vi "VI Data Extractor.vi"(7 "Port number":u16=3364, 8 "error in (no error)":errorcluster, 10 "Output path":path, 11 "VI Path":path) -> (0 "error out":errorcluster, 3 "path":path)   [LabVIEW 2024]
uses:
  <vilib>/Utility/traverseref.llb/TRef TravTarget.ctl
  <vilib>/Utility/miscctls.llb/LVPositionTypeDef.ctl
  <vilib>/Utility/miscctls.llb/LVBoundsTypeDef.ctl
  <vilib>/Utility/miscctls.llb/LVMapReplaceAction.ctl
  <vilib>/Utility/traverseref.llb/VI Scripting - Traverse.lvlib
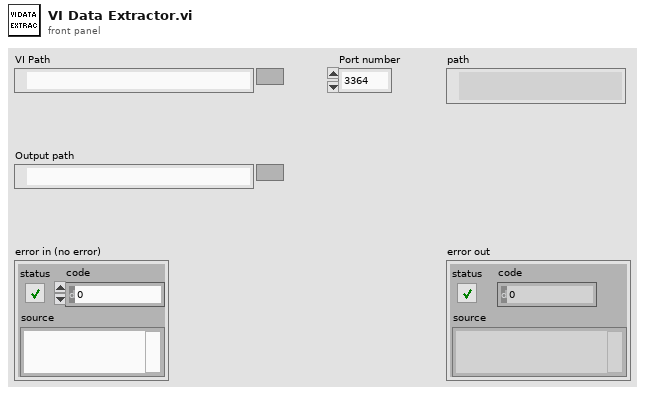
[diagram p1: front panel]
types:
  T1 = typedef "LVPositionTypeDef.ctl" = cluster{"Left":i32, "Top":i32}
  T2 = typedef "LVBoundsTypeDef.ctl" = cluster{"Width":u32, "Height":u32}
  T3 = map{i32, cluster{"Diagram Data":cluster{"UID":i32, "Diagram Image":string}[], "Position":T1, "Bounds":T2, "Is on TLD?":bool}}
  T4 = cluster{"TLD Position":T1, "TLD":string, "Structure to Diagram":cluster{"UID":i32, "Diagram Group":cluster{"Diagram Data":cluster{"UID":i32, "Diagram Image":string}[], "Position":T1, "Bounds":T2, "Is on TLD?":bool}}[], "Diagram to Structure":cluster{"Diagram UID":i32, "Diagram Children":i32[]}[], "BD Color":string, "TLD Bounds":T2}
  T5 = typedef "TRef TravTarget.ctl" = enum16{"FP", "BD", "Other"}
  T6 = typedef "imagedata.ctl" = cluster{"image type":i32, "image depth":i32, "image":u8[], "mask":u8[], "colors":u32[], "Rectangle":cluster{"left":i16, "top":i16, "right":i16, "bottom":i16}}
  T7 = cluster{"Diagram Data":cluster{"UID":i32, "Diagram Image":string}[], "Position":T1, "Bounds":T2, "Is on TLD?":bool}
  T8 = typedef "LVMapReplaceAction.ctl" = enum32{"Modify Entry only if found", "Add or Modify Entry", "Delete Entry"}
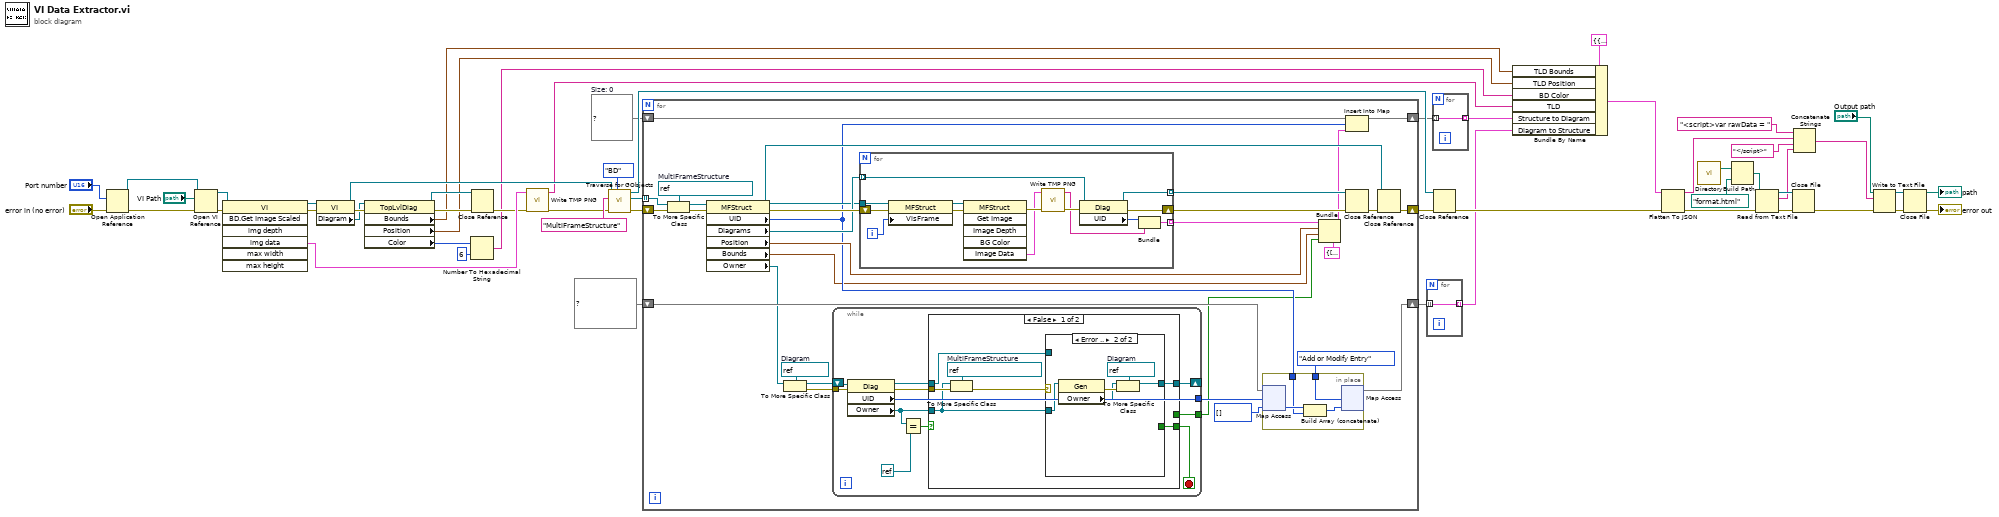
[diagram p0: block diagram]
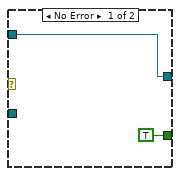
[diagram p2: hidden frame]
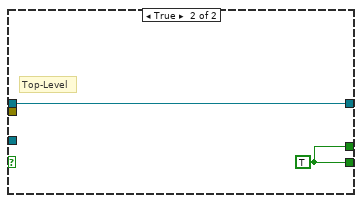
[diagram p3: hidden frame]
diagram:
  w30 = T3 {}  # Size: 0
  n1 = Open Application Reference(8:"error in (no error)", 10:"Port number") -> (0:w15:errorcluster, 3:w13:refnum<vi>)  [unwired: 2 in]
  n2 = Open VI Reference(application reference (local)=w13, vi path="VI Path", error in (no error)=w15) -> (vi reference=w6:refnum<vi>, error out=w16:errorcluster)  [unwired: 3 in]
  n3 = invoke class="VI" method="BD.Get Image Scaled"(reference=w6, error in=w16) -> (reference out=w40:refnum<vi>, error out=w41:errorcluster, "img data"=w49:T6)  [unwired: 5 in, 4 out]
  n4 = property class="VI"(reference=w40, error in=w41) -> (reference out=w39:refnum<vi>, error out=w38:errorcluster, "Diagram"=w37:refnum<vi>)
  n5 = property class="TopLvlDiag"(reference=w37, error in=w38) -> (reference out=w34:refnum<vi>, error out=w36:errorcluster, "Bounds"=w1:T2, "Position"=w3:T1, "Color"=w4:u32)
  n6 = Number To Hexadecimal String(1:i16 6 ("width (-)"), 2:w4) -> (0:w2:string)
  n7 = Close Reference(reference=w34, error in (no error)=w36) -> (error out=w35:errorcluster)
  n8 = call "Write TMP PNG.vi"("error in (no error)"=w35, "img data"=w49) -> ("error out"=w50:errorcluster, "Base64 Encoded"=w33:string)  [unwired: 8 in]
  n9 = call <vilib>:"Traverse for GObjects.vi"("Traverse Target"=TRef_TravTarget."BD", "error in (no error)"=w50, "Class Name"="MultiFrameStructure", "VI Refnum"=w39) -> ("error out"=w52:errorcluster, "References"=w51:refnum<vi>[], "dup VI Refnum"=w47:refnum<vi>)  [unwired: 4 in, 1 out]
  n10 = for {
    tunnel: w51 -> [w84] mode=indexing
    shift-right: [w77] -> w46
    shift-left: w30 -> [w78]
    shift-right: [w73] -> w48
    shift-left: w52 -> [w85]
    shift-right: [w65] -> w44
    shift-left: map{i32, i32[]} {} ("Map") -> [w66]
    w59 = refnum<vi> refnum  # Diagram
    w81 = refnum<vi> refnum  # MultiFrameStructure
    n11 = To More Specific Class(target class=w81, reference=w84, error in=w85) -> (specific class reference=w82:refnum<vi>, error out=w83:errorcluster)
    n12 = property class="MFStruct"(reference=w82, error in=w83) -> (reference out=w72:refnum<vi>, error out=w80:errorcluster, "UID"=w63:i32, "Diagrams"=w79:refnum<vi>[], "Position"=w71:T1, "Bounds"=w60:T2, "Owner"=w58:refnum<vi>)
    n13 = To More Specific Class(target class=w59, reference=w58) -> (specific class reference=w57:refnum<vi>, error out=w56:errorcluster)  [unwired: 1 in]
    n14 = while {
      tunnel: [w96] -> w68
      tunnel: [w90] -> w61
      tunnel: w56 -> [w92]
      shift-right: [w89] -> _
      shift-left: w57 -> [w93]
      stop <- w91 stop-if-true
      n15 = property class="Diag"(reference=w93, error in=w92) -> (reference out=w86:refnum<vi>, error out=w87:errorcluster, "UID"=w96:i32, "Owner"=w88:refnum<vi>)
      n16 = Equal?(x=w88, y=refnum<k0> refnum) -> (x = y?=w94:bool)
      n17 = case shown="False" w94 {
        tunnel: [w100 w112] -> w91
        tunnel: [_ w112] -> w90
        tunnel: [w98 w111] -> w89
        tunnel: w88 -> [w99 _]
        tunnel: w87 -> [w102 _]
        tunnel: w86 -> [w97 w111]
        frame False {
          w103 = refnum<vi> refnum  # MultiFrameStructure
          n18 = To More Specific Class(target class=w103, reference=w99, error in=w102) -> (error out=w101:errorcluster)  [unwired: 1 out]
          n19 = case shown="Error .." w101 {
            tunnel: [TRUE ("Boolean") _] -> w100
            tunnel: w99 -> [_ w110]
            tunnel: [w104 w107] -> w98
            tunnel: w97 -> [w104 _]
            frame No Error {
            }
            frame Error {
              w109 = refnum<vi> refnum  # Diagram
              n20 = property class="Gen"(reference=w110) -> (error out=w108:errorcluster, "Owner"=w106:refnum<vi>)  [unwired: 1 in, 1 out]
              n21 = To More Specific Class(target class=w109, reference=w106, error in=w108) -> (specific class reference=w107:refnum<vi>)  [unwired: 1 out]
            }
          }
        }
        frame True {
          w112 = TRUE ("Boolean")
          # "Top-Level"
        }
      }
    }
    n22 = for {
      tunnel: w79 -> [w130] mode=indexing
      tunnel: [w121] -> w70 mode=indexing
      shift-right: [w129] -> w76
      shift-left: w80 -> [w127]
      tunnel: [w128] -> w75 mode=indexing
      tunnel: w72 -> [w126]
      i -> [w125]
      n23 = property class="MFStruct"(reference=w126, error in=w127, "VisFrame"=w125) -> (reference out=w123:refnum<vi>, error out=w124:errorcluster)
      n24 = invoke class="MFStruct" method="Get Image"(reference=w123, error in=w124) -> (error out=w120:errorcluster, "Image Data"=w118:T6)  [unwired: 4 in, 4 out]
      n25 = call "Write TMP PNG.vi"("error in (no error)"=w120, "img data"=w118) -> ("error out"=w119:errorcluster, "Base64 Encoded"=w117:string)  [unwired: 8 in]
      n26 = property class="Diag"(reference=w130, error in=w119) -> (reference out=w128:refnum<vi>, error out=w129:errorcluster, "UID"=w122:i32)
      n27 = Bundle("UID"=w122, "Base64 Encoded"=w117) -> (w121:cluster{"UID":i32, "Base64 Encoded":string})  [unwired: 1 in]
    }
    n28 = in-place {
      in-place-border: LVMapReplaceAction."Add or Modify Entry" ("Replace Action") -> [w114]
      in-place-border: w63 -> [w113]
      n29 = in-place-map #1(w66, w68, i32[] [] ("output cluster")) -> (w116:i32[])  [unwired: 1 out]
      n30 = Build Array (concatenate)(w116, w113) -> (w115:i32[])
      n31 = in-place-map #1(w115, w114) -> (w65:map{i32, i32[]})  [unwired: 2 out]
    }
    n32 = Bundle(cluster=T7 {"Diagram Data"=[], "Position"={"Left"=0, "Top"=0}, "Bounds"={"Width"=0, "Height"=0}, "Is on TLD?"=FALSE} ("Diagram Group"), "Diagram Data"=w70, "Position"=w71, "Bounds"=w60, "Is on TLD?"=w61) -> (w69:T7)
    n33 = Insert Into Map(map in=w78, key=w63, value=w69) -> (map out=w77:T3)  [unwired: 2 out]
    n34 = Close Reference(reference=w75, error in (no error)=w76) -> (error out=w74:errorcluster)
    n35 = Close Reference(reference=w72, error in (no error)=w74) -> (error out=w73:errorcluster)
  }
  n36 = for {
    tunnel: w44 -> [w131] mode=indexing
    tunnel: [w131] -> w31 mode=indexing
  }
  n37 = for {
    tunnel: w46 -> [w132] mode=indexing
    tunnel: [w132] -> w32 mode=indexing
  }
  n38 = Close Reference(reference=w47, error in (no error)=w48) -> (error out=w43:errorcluster)
  n39 = Bundle By Name(cluster=T4 {"TLD Position"={"Left"=0, "Top"=0}, "TLD"="", "Structure to Diagram"=[], "Diagram to Structure"=[], "BD Color"="", "TLD Bounds"={"Width"=0, "Height"=0}}, "TLD Bounds"=w1, "TLD Position"=w3, "BD Color"=w2, "TLD"=w33, "Structure to Diagram"=w32, "Diagram to Structure"=w31) -> (w45:T4)
  n40 = Flatten To JSON(anything=w45, error in (no error)=w43) -> (JSON string=w24:string, 11:w8:errorcluster)  [unwired: 1 in]
  n41 = call "Directory.vi"() -> ("Directory"=w7:path)  [unwired: 3 in]
  n42 = Build Path(base path=w7, name or relative path=path "format.html") -> (appended path=w27:path)
  n43 = Read from Text File(file (use dialog)=w27, error in=w8) -> (refnum out=w26:refnum<file>, text=w9:string, error out=w25:errorcluster)  [unwired: 2 in, 1 out]
  n44 = Close File(refnum=w26, error in=w25) -> (error out=w11:errorcluster)  [unwired: 1 out]
  n45 = Concatenate Strings("<script>var rawData = " ("string"), w24, "</script>" ("string"), w9) -> (w21:string)
  n46 = Write to Text File(file (use dialog)="Output path", text=w21, error in=w11) -> (refnum out=w20:refnum<file>, error out=w19:errorcluster)  [unwired: 1 in, 1 out]
  n47 = Close File(refnum=w20, error in=w19) -> (path=→"path":path, error out=→"error out":errorcluster)
